vi "Accelerometer.vi"() -> ()   [LabVIEW 2021]
uses:
  <vilib>/Math Plots/3D Math Plots/3D Scatter/3D Scatter XCtrl/3D Scatter.xctl
  <vilib>/Math Plots/3D Math Plots/3D Scatter/3D Scatter Datatype/3D Scatter Datatype.lvclass
  <vilib>/DAQmx/read.llb/DAQmx Read (Analog 1D Wfm NChan NSamp).vi
  <vilib>/DAQmx/create/channels.llb/DAQmx Create Channel (AI-Voltage-Basic).vi
  <vilib>/DAQmx/configure/timing.llb/DAQmx Timing (Sample Clock).vi
  <vilib>/DAQmx/miscellaneous.llb/DAQmx Fill In Error Info.vi
  <vilib>/Utility/file.llb/Read Delimited Spreadsheet (DBL).vi
  <vilib>/Math Plots/3D Math Plots/3D Scatter/3D Scatter Datatype/Public/Plot Helper (Matrices).vi
  <vilib>/Utility/file.llb/Write Delimited Spreadsheet (DBL).vi
  <resource>/objmgr/daqmx.rc
  <vilib>/ptbypt/NI_PtbyPt.lvlib
  <vilib>/Analysis/NI_AALPro.lvlib
panel:
  out "VOLTAGE Z":dbl=-1.4400705579380926 format="%#_13g"
  in  "STOP ALL":bool
  in  "timeout":dbl=10.0 format="%0.2f"
  out "VOLTAGE Y":dbl=-1.6616253135787673 format="%#_13g"
  out "VOLTAGE X":dbl=1.114440988590271 format="%#_13g"
  out "3-Signal Waveform":waveform(dbl)[](graph)=[{"t0"=timestamp(3794378282.2177434 s since 1904-01-01), "dt"=0.001, "Y"=[1.02776641981038, 1.0481604359938839, 1.02776641981038, 1.1195394926361484, 1.1093424845443955, 1.1297365007278994, 1.1195394926361484, 1.134835004773775, 1.0991454764526445, 1.0991454764526445, 1.1705245330949072, 1.1909185492784111, 1.1654260290490317, 1.1705245330949072, 1.211312565461915, 1.1858200452325356, 1.1756230371407845, 1.1297365007278994, 1.0889484683608917, 1.0736529562232633, 0.9818798833974949, 1.0022738995809988, 1.0481604359938839, 1.114440988590271, 1.1399335088196523, 1.134835004773775, 1.1195394926361484, 1.124637996682024, 1.134835004773775, 1.0838499643150161, 1.124637996682024, 1.1450320128655278, 1.1399335088196523, 1.1603275250031562, 1.1093424845443955, 1.1501305169114033, 1.1858200452325356, 1.1399335088196523, 1.1450320128655278, 1.1450320128655278, 1.1501305169114033, 1.201115557370164, 1.201115557370164, 1.1399335088196523, 1.0991454764526445, 1.0991454764526445, 1.0940469724067672, 1.0991454764526445, 1.0838499643150161, 1.1195394926361484, 1.1195394926361484, 1.1399335088196523, 1.1552290209572806, 1.1705245330949072, 1.0991454764526445, 1.1399335088196523, 1.1501305169114033, 1.10424398049852, 1.0481604359938839, 1.0736529562232633, 1.1093424845443955, 1.1297365007278994, 1.0838499643150161, 1.058357444085635, 1.0481604359938839, 1.0532589400397594, 1.0736529562232633, 1.1195394926361484, 1.124637996682024, 1.10424398049852, 1.1399335088196523, 1.134835004773775, 1.1705245330949072, 1.1399335088196523, 1.2062140614160395, 1.1909185492784111, 1.1705245330949072, 1.1399335088196523, 1.0838499643150161, 1.124637996682024, 1.1195394926361484, 1.134835004773775, 1.0787514602691388, 1.114440988590271, 1.1399335088196523, 1.114440988590271, 1.1297365007278994, 1.0991454764526445, 1.1501305169114033, 1.134835004773775, 1.124637996682024, 1.0736529562232633, 1.0991454764526445, 1.1450320128655278, 1.1297365007278994, 1.1756230371407845, 1.1450320128655278, 1.1450320128655278, 1.114440988590271, 1.114440988590271], "attributes"=variant("NI_ChannelName"=variant(string "Dev1/ai0"), "NI_UnitDescription"=variant(string "Volts"))}, {"t0"=timestamp(3794378282.217764 s since 1904-01-01), "dt"=0.001, "Y"=[-1.6157110871262397, -1.6514221521448729, -1.6463205714279248, -1.6412189907109767, -1.6412189907109767, -1.6106095064092916, -1.6106095064092916, -1.5800000221076065, -1.5544921185228695, -1.564695279956764, -1.6055079256923452, -1.6412189907109767, -1.6412189907109767, -1.6055079256923452, -1.6106095064092916, -1.6004063449753971, -1.6055079256923452, -1.6157110871262397, -1.6208126678431878, -1.6259142485601341, -1.6004063449753971, -1.564695279956764, -1.595304764258449, -1.6412189907109767, -1.6616253135787673, -1.6463205714279248, -1.6259142485601341, -1.6055079256923452, -1.5800000221076065, -1.595304764258449, -1.5493905378059214, -1.6718284750126635, -1.6514221521448729, -1.6463205714279248, -1.6361174099940303, -1.6514221521448729, -1.73814902433298, -1.7024379593143486, -1.6973363785974005, -1.682031636446558, -1.6922347978804524, -1.6463205714279248, -1.6667268942957154, -1.6973363785974005, -1.687133217163506, -1.6769300557296098, -1.6004063449753971, -1.5851016028245546, -1.682031636446558, -1.6310158292770822, -1.595304764258449, -1.6208126678431878, -1.6106095064092916, -1.6412189907109767, -1.6106095064092916, -1.595304764258449, -1.6259142485601341, -1.6616253135787673, -1.6922347978804524, -1.6616253135787673, -1.6463205714279248, -1.687133217163506, -1.6973363785974005, -1.6769300557296098, -1.656523732861821, -1.6514221521448729, -1.6259142485601341, -1.5851016028245546, -1.6208126678431878, -1.6463205714279248, -1.595304764258449, -1.6259142485601341, -1.6922347978804524, -1.707539540031295, -1.712641120748243, -1.6667268942957154, -1.6973363785974005, -1.682031636446558, -1.7177427014651911, -1.6718284750126635, -1.687133217163506, -1.7432506050499281, -1.73814902433298, -1.6973363785974005, -1.6973363785974005, -1.682031636446558, -1.6514221521448729, -1.6361174099940303, -1.5851016028245546, -1.6208126678431878, -1.5800000221076065, -1.595304764258449, -1.6106095064092916, -1.569796860673712, -1.5851016028245546, -1.564695279956764, -1.5748984413906602, -1.6004063449753971, -1.6514221521448729, -1.6616253135787673], "attributes"=variant("NI_ChannelName"=variant(string "Dev1/ai1"), "NI_UnitDescription"=variant(string "Volts"))}, {"t0"=timestamp(3794378282.217785 s since 1904-01-01), "dt"=0.001, "Y"=[-1.3533473747749927, -1.3584487384904698, -1.3788541933523764, -1.3329419199130879, -1.2972323739047518, -1.307435101335706, -1.2972323739047518, -1.276826919042847, -1.3329419199130879, -1.3788541933523764, -1.3890569207833288, -1.3023337376202289, -1.338043283628565, -1.4400705579380926, -1.4400705579380926, -1.4400705579380926, -1.4400705579380926, -1.4247664667916649, -1.3992596482142812, -1.4196651030761878, -1.4604760127999992, -1.5063882862392877, -1.4910841950928582, -1.4655773765154763, -1.485982831377381, -1.4961855588083353, -1.455374649084522, -1.3890569207833288, -1.3329419199130879, -1.3788541933523764, -1.3788541933523764, -1.4808814676619058, -1.3584487384904698, -1.3431446473440403, -1.3533473747749927, -1.2717255553273699, -1.2411173730345109, -1.338043283628565, -1.3839555570678517, -1.338043283628565, -1.4451719216535697, -1.3941582844988059, -1.338043283628565, -1.4196651030761878, -1.4349691942226173, -1.3737528296368993, -1.3584487384904698, -1.3176378287666584, -1.4910841950928582, -1.3992596482142812, -1.3176378287666584, -1.3584487384904698, -1.2564214641809404, -1.3533473747749927, -1.3635501022059469, -1.3329419199130879, -1.338043283628565, -1.3635501022059469, -1.3584487384904698, -1.3584487384904698, -1.3125364650511813, -1.307435101335706, -1.3278405561976108, -1.3737528296368993, -1.3890569207833288, -1.338043283628565, -1.3125364650511813, -1.3533473747749927, -1.4298678305071402, -1.4604760127999992, -1.3992596482142812, -1.4349691942226173, -1.3737528296368993, -1.3941582844988059, -1.4094623756452354, -1.4298678305071402, -1.4757801039464287, -1.455374649084522, -1.4961855588083353, -1.4400705579380926, -1.4604760127999992, -1.4808814676619058, -1.5012869225238106, -1.4451719216535697, -1.5012869225238106, -1.5523005596785762, -1.4655773765154763, -1.3890569207833288, -1.3737528296368993, -1.4808814676619058, -1.4655773765154763, -1.5676046508250057, -1.4706787402309516, -1.485982831377381, -1.4094623756452354, -1.3737528296368993, -1.4043610119297583, -1.4451719216535697, -1.4400705579380926, -1.4400705579380926], "attributes"=variant("NI_ChannelName"=variant(string "Dev1/ai2"), "NI_UnitDescription"=variant(string "Volts"))}]
  out "Z-Signal Waveform":dynamicdata(graph)=[{"t0"=timestamp(3794378282.217785 s since 1904-01-01), "dt"=0.001, "Y"=[-1.3533473747749927, -1.3584487384904698, -1.3788541933523764, -1.3329419199130879, -1.2972323739047518, -1.307435101335706, -1.2972323739047518, -1.276826919042847, -1.3329419199130879, -1.3788541933523764, -1.3890569207833288, -1.3023337376202289, -1.338043283628565, -1.4400705579380926, -1.4400705579380926, -1.4400705579380926, -1.4400705579380926, -1.4247664667916649, -1.3992596482142812, -1.4196651030761878, -1.4604760127999992, -1.5063882862392877, -1.4910841950928582, -1.4655773765154763, -1.485982831377381, -1.4961855588083353, -1.455374649084522, -1.3890569207833288, -1.3329419199130879, -1.3788541933523764, -1.3788541933523764, -1.4808814676619058, -1.3584487384904698, -1.3431446473440403, -1.3533473747749927, -1.2717255553273699, -1.2411173730345109, -1.338043283628565, -1.3839555570678517, -1.338043283628565, -1.4451719216535697, -1.3941582844988059, -1.338043283628565, -1.4196651030761878, -1.4349691942226173, -1.3737528296368993, -1.3584487384904698, -1.3176378287666584, -1.4910841950928582, -1.3992596482142812, -1.3176378287666584, -1.3584487384904698, -1.2564214641809404, -1.3533473747749927, -1.3635501022059469, -1.3329419199130879, -1.338043283628565, -1.3635501022059469, -1.3584487384904698, -1.3584487384904698, -1.3125364650511813, -1.307435101335706, -1.3278405561976108, -1.3737528296368993, -1.3890569207833288, -1.338043283628565, -1.3125364650511813, -1.3533473747749927, -1.4298678305071402, -1.4604760127999992, -1.3992596482142812, -1.4349691942226173, -1.3737528296368993, -1.3941582844988059, -1.4094623756452354, -1.4298678305071402, -1.4757801039464287, -1.455374649084522, -1.4961855588083353, -1.4400705579380926, -1.4604760127999992, -1.4808814676619058, -1.5012869225238106, -1.4451719216535697, -1.5012869225238106, -1.5523005596785762, -1.4655773765154763, -1.3890569207833288, -1.3737528296368993, -1.4808814676619058, -1.4655773765154763, -1.5676046508250057, -1.4706787402309516, -1.485982831377381, -1.4094623756452354, -1.3737528296368993, -1.4043610119297583, -1.4451719216535697, -1.4400705579380926, -1.4400705579380926], "attributes"=variant("NI_ChannelName"=variant(string "Dev1/ai2"), "NI_UnitDescription"=variant(string "Volts"))}]
  out "Y-Signal Waveform":dynamicdata(graph)=[{"t0"=timestamp(3794378282.217764 s since 1904-01-01), "dt"=0.001, "Y"=[-1.6157110871262397, -1.6514221521448729, -1.6463205714279248, -1.6412189907109767, -1.6412189907109767, -1.6106095064092916, -1.6106095064092916, -1.5800000221076065, -1.5544921185228695, -1.564695279956764, -1.6055079256923452, -1.6412189907109767, -1.6412189907109767, -1.6055079256923452, -1.6106095064092916, -1.6004063449753971, -1.6055079256923452, -1.6157110871262397, -1.6208126678431878, -1.6259142485601341, -1.6004063449753971, -1.564695279956764, -1.595304764258449, -1.6412189907109767, -1.6616253135787673, -1.6463205714279248, -1.6259142485601341, -1.6055079256923452, -1.5800000221076065, -1.595304764258449, -1.5493905378059214, -1.6718284750126635, -1.6514221521448729, -1.6463205714279248, -1.6361174099940303, -1.6514221521448729, -1.73814902433298, -1.7024379593143486, -1.6973363785974005, -1.682031636446558, -1.6922347978804524, -1.6463205714279248, -1.6667268942957154, -1.6973363785974005, -1.687133217163506, -1.6769300557296098, -1.6004063449753971, -1.5851016028245546, -1.682031636446558, -1.6310158292770822, -1.595304764258449, -1.6208126678431878, -1.6106095064092916, -1.6412189907109767, -1.6106095064092916, -1.595304764258449, -1.6259142485601341, -1.6616253135787673, -1.6922347978804524, -1.6616253135787673, -1.6463205714279248, -1.687133217163506, -1.6973363785974005, -1.6769300557296098, -1.656523732861821, -1.6514221521448729, -1.6259142485601341, -1.5851016028245546, -1.6208126678431878, -1.6463205714279248, -1.595304764258449, -1.6259142485601341, -1.6922347978804524, -1.707539540031295, -1.712641120748243, -1.6667268942957154, -1.6973363785974005, -1.682031636446558, -1.7177427014651911, -1.6718284750126635, -1.687133217163506, -1.7432506050499281, -1.73814902433298, -1.6973363785974005, -1.6973363785974005, -1.682031636446558, -1.6514221521448729, -1.6361174099940303, -1.5851016028245546, -1.6208126678431878, -1.5800000221076065, -1.595304764258449, -1.6106095064092916, -1.569796860673712, -1.5851016028245546, -1.564695279956764, -1.5748984413906602, -1.6004063449753971, -1.6514221521448729, -1.6616253135787673], "attributes"=variant("NI_ChannelName"=variant(string "Dev1/ai1"), "NI_UnitDescription"=variant(string "Volts"))}]
  out "X-Signal Waveform":dynamicdata(graph)=[{"t0"=timestamp(3794378282.2177434 s since 1904-01-01), "dt"=0.001, "Y"=[1.02776641981038, 1.0481604359938839, 1.02776641981038, 1.1195394926361484, 1.1093424845443955, 1.1297365007278994, 1.1195394926361484, 1.134835004773775, 1.0991454764526445, 1.0991454764526445, 1.1705245330949072, 1.1909185492784111, 1.1654260290490317, 1.1705245330949072, 1.211312565461915, 1.1858200452325356, 1.1756230371407845, 1.1297365007278994, 1.0889484683608917, 1.0736529562232633, 0.9818798833974949, 1.0022738995809988, 1.0481604359938839, 1.114440988590271, 1.1399335088196523, 1.134835004773775, 1.1195394926361484, 1.124637996682024, 1.134835004773775, 1.0838499643150161, 1.124637996682024, 1.1450320128655278, 1.1399335088196523, 1.1603275250031562, 1.1093424845443955, 1.1501305169114033, 1.1858200452325356, 1.1399335088196523, 1.1450320128655278, 1.1450320128655278, 1.1501305169114033, 1.201115557370164, 1.201115557370164, 1.1399335088196523, 1.0991454764526445, 1.0991454764526445, 1.0940469724067672, 1.0991454764526445, 1.0838499643150161, 1.1195394926361484, 1.1195394926361484, 1.1399335088196523, 1.1552290209572806, 1.1705245330949072, 1.0991454764526445, 1.1399335088196523, 1.1501305169114033, 1.10424398049852, 1.0481604359938839, 1.0736529562232633, 1.1093424845443955, 1.1297365007278994, 1.0838499643150161, 1.058357444085635, 1.0481604359938839, 1.0532589400397594, 1.0736529562232633, 1.1195394926361484, 1.124637996682024, 1.10424398049852, 1.1399335088196523, 1.134835004773775, 1.1705245330949072, 1.1399335088196523, 1.2062140614160395, 1.1909185492784111, 1.1705245330949072, 1.1399335088196523, 1.0838499643150161, 1.124637996682024, 1.1195394926361484, 1.134835004773775, 1.0787514602691388, 1.114440988590271, 1.1399335088196523, 1.114440988590271, 1.1297365007278994, 1.0991454764526445, 1.1501305169114033, 1.134835004773775, 1.124637996682024, 1.0736529562232633, 1.0991454764526445, 1.1450320128655278, 1.1297365007278994, 1.1756230371407845, 1.1450320128655278, 1.1450320128655278, 1.114440988590271, 1.114440988590271], "attributes"=variant("NI_ChannelName"=variant(string "Dev1/ai0"), "NI_UnitDescription"=variant(string "Volts"))}]
  out "SampClk.Rate":dbl=1000.0
  in  "Modalità di campionamento":i32(ring)=10123 items=["Finite Samples"=10178, "Continuous Samples"=10123, "Hardware Timed Single Point"=12522]
  in  "Campioni per canale":i32=100
  in  "Rate":dbl=1000.0 format="%0.2f"
  in  "Canale Fisico":tag="Dev1/ai0:2"
  in  "MIN Value":dbl=-10.0 format="%0.2f"
  in  "MAX Value":dbl=10.0 format="%0.2f"
  in  "Tab Control":T1(tab)=enum."CALIBRATION"
  in  "File z":path=path "C:/Users/Engel/Desktop/MAIP_Project/Z.csv"
  in  "File y":path=path "C:/Users/Engel/Desktop/MAIP_Project/Y.csv"
  in  "File x":path=path "C:/Users/Engel/Desktop/MAIP_Project/X.csv"
  in  "Salvare su file?":bool=TRUE
  out "Real values":refnum<class "3D Plot Datatype.lvclass">[](xcontrol)
  in  "Usare il filtro a\n media mobile?":bool
  out "h":dbl[][](array[numeric])
  in  "Z":path=path "C:/Users/Engel/Documents/Dati_ellisse/dati_buoni_BRACCIO/Z.csv"
  in  "X":path=path "C:/Users/Engel/Documents/Dati_ellisse/dati_buoni_BRACCIO/X.csv"
  in  "Y":path=path "C:/Users/Engel/Documents/Dati_ellisse/dati_buoni_BRACCIO/Y.csv"
  out "Real values 2":refnum<class "3D Plot Datatype.lvclass">[](xcontrol)
  out "Best Linear Fit":dbl[](array[numeric])=[-90.70772285582407, 1.4505193173588147, 89.25720353846528]
  in  "Tensioni":path=path "C:/Users/Engel/Desktop/Dati/Z TAR/mean_z.txt"
  in  "Gradi":path=path "C:/Users/Engel/Desktop/Dati/Gradi6/Gradi.txt"
  out "Gradi\nz":dbl[](array[numeric])=[-91.51190382332419]
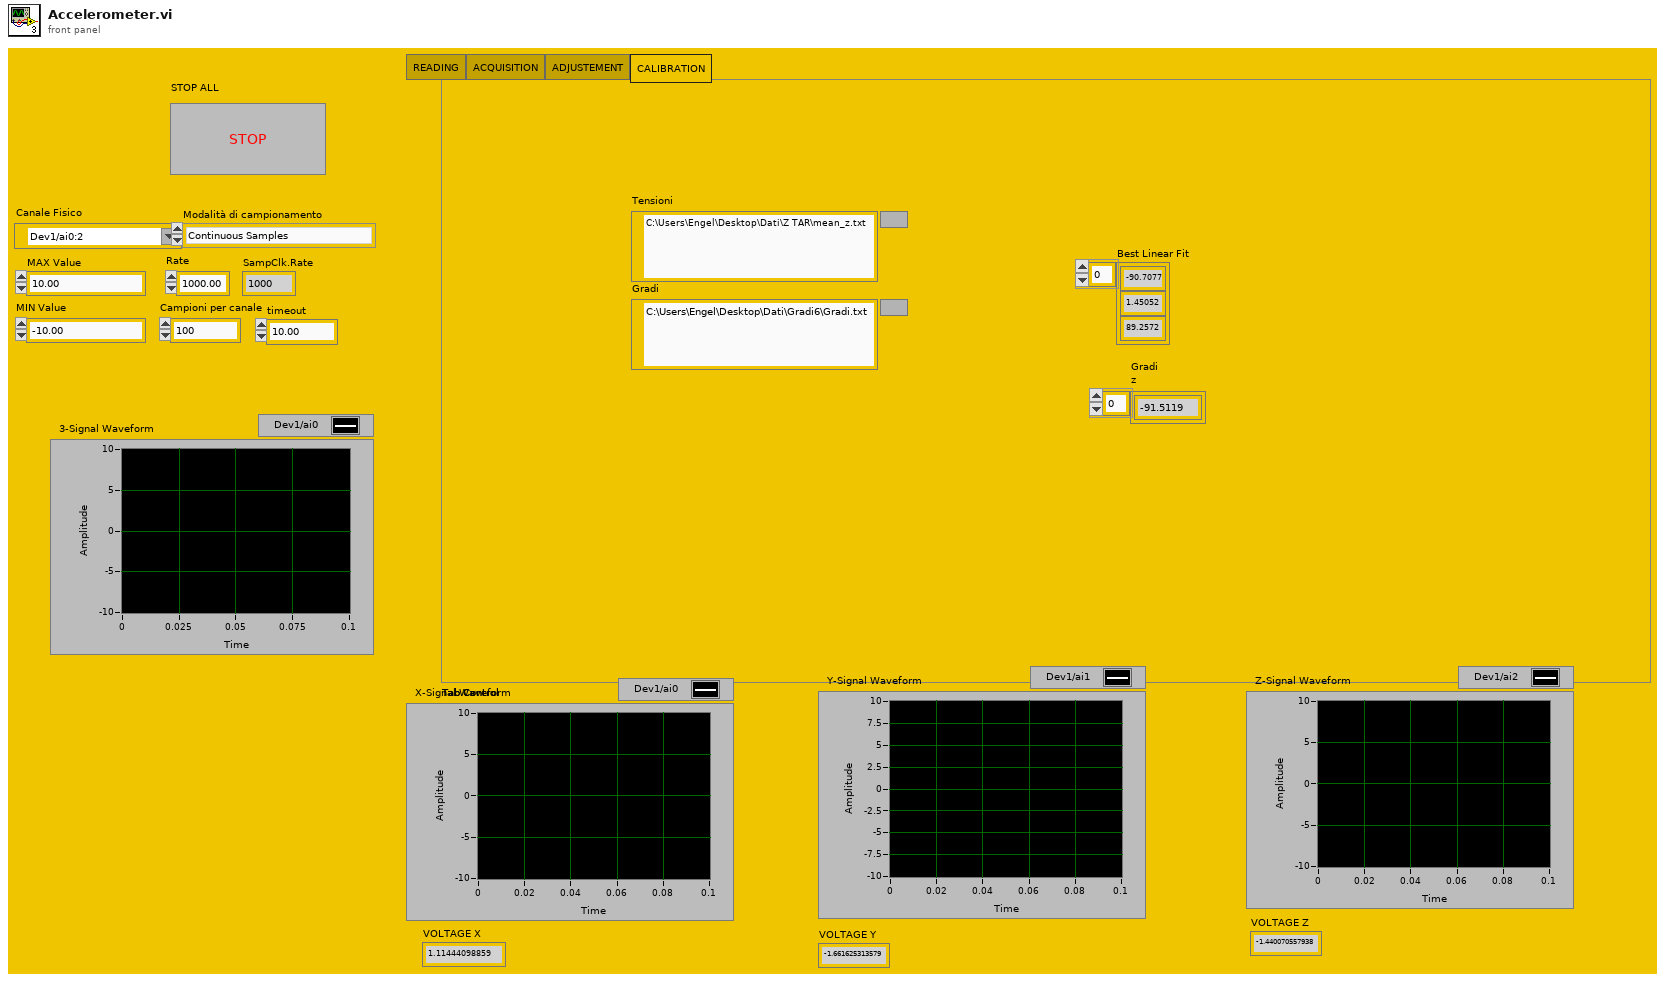
[diagram p1: front panel]
types:
  T1 = enum32{"READING", "ACQUISITION", "ADJUSTEMENT", "CALIBRATION"}
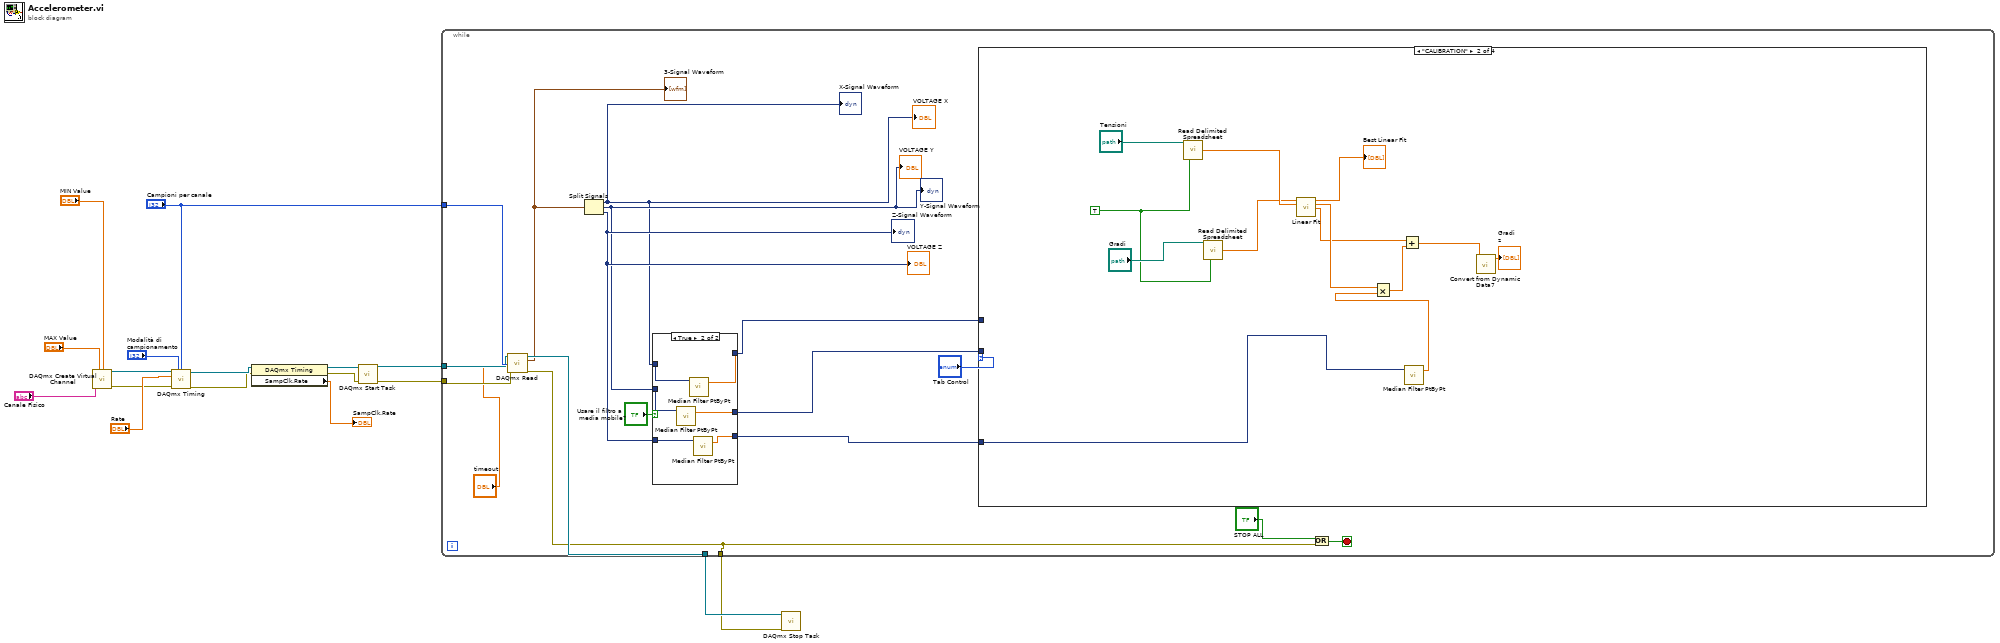
[diagram p0: block diagram]
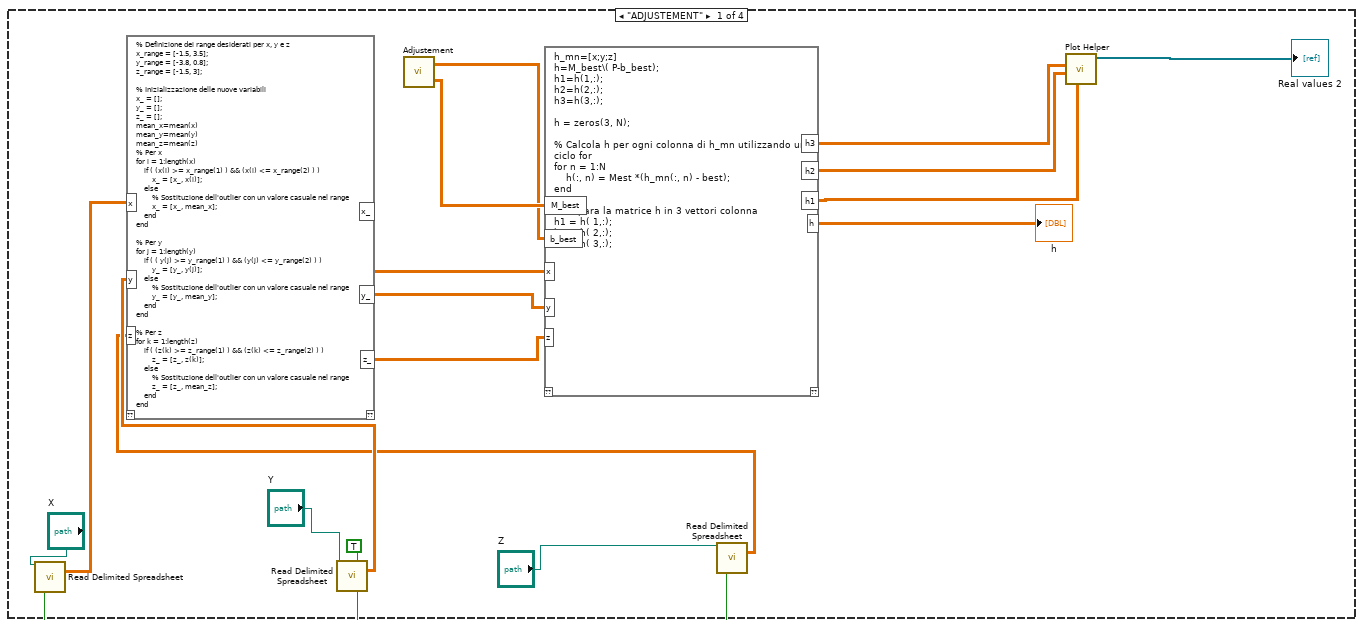
[diagram p3: hidden frame]
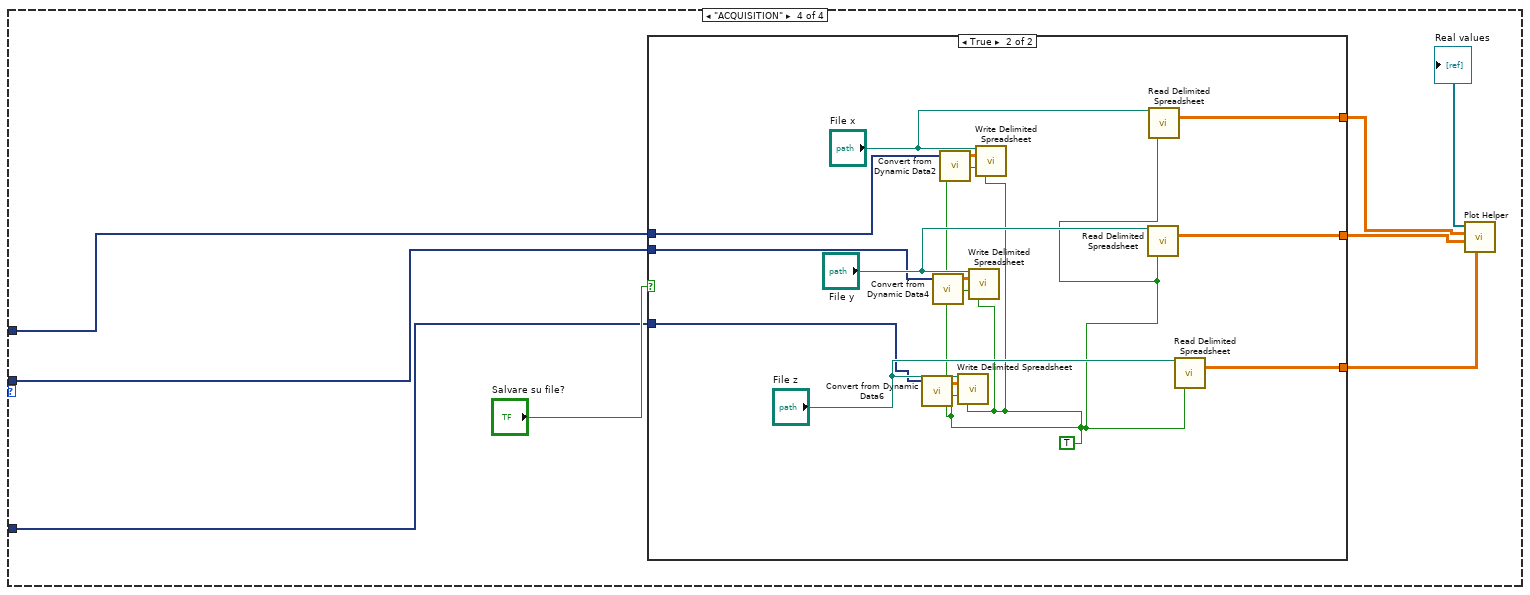
[diagram p5: hidden frame]
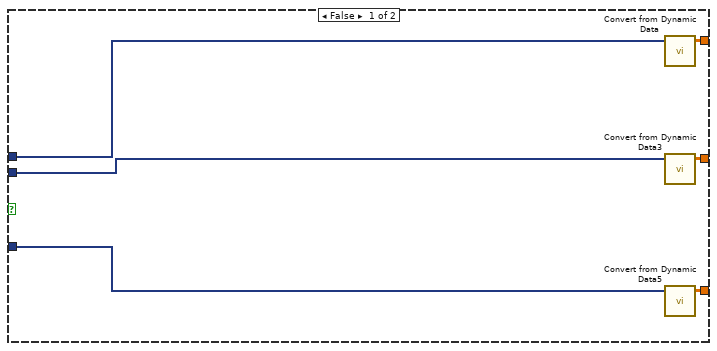
[diagram p6: hidden frame]
diagram:
  n1 = call-poly <vilib>:"DAQmx Create Virtual Channel.vi"("maximum value"="MAX Value", "minimum value"="MIN Value", "physical channels"="Canale Fisico") -> ("task out"=w14:refnum<k21>, "error out"=w11:errorcluster)  [unwired: 11 in]
  n2 = call-poly <vilib>:"DAQmx Timing.vi"("task/channels in"=w14, "sample mode"="Modalità di campionamento", "samples per channel"="Campioni per canale", "rate"="Rate", "error in"=w11) -> ("task out"=w9:refnum<k21>, "error out"=w8:errorcluster)  [unwired: 9 in]
  n3 = property class="DAQmx Timing"(reference=w9, error in=w8) -> (reference out=w7:refnum<k21>, error out=w6:errorcluster, "SampClk.Rate"=→"SampClk.Rate":dbl)
  n4 = call <vilib>:"DAQmx Start Task.vi"("task/channels in"=w7, "error in"=w6) -> ("task out"=w5:refnum<k21>, "error out"=w3:errorcluster)  [unwired: 12 in]
  n5 = while {
    tunnel: w5 -> [w30]
    tunnel: "Campioni per canale" -> [w31]
    tunnel: w3 -> [w29]
    tunnel: [w28] -> w2
    tunnel: [w27] -> w1
    stop <- w32 stop-if-true
    n6 = call-poly <vilib>:"DAQmx Read.vi"("task/channels in"=w30, "number of samples per channel"=w31, "timeout"="timeout", "error in"=w29) -> ("task out"=w28:refnum<k21>, "data"=w26:waveform(dbl)[], "error out"=w27:errorcluster)  [unwired: 9 in]
    "3-Signal Waveform" <- w26
    n7 = Split Signals(w26) -> (w20:dynamicdata, w22:dynamicdata, w24:dynamicdata)  [unwired: 3 in]
    "Z-Signal Waveform" <- w24
    "Y-Signal Waveform" <- w22
    "X-Signal Waveform" <- w20
    "VOLTAGE X" <- w20
    "VOLTAGE Y" <- w22
    "VOLTAGE Z" <- w24
    n8 = case shown="True" "Usare il filtro a\n media mobile?" {
      tunnel: w24 -> [w35 w43]
      tunnel: [w35 w42] -> w23
      tunnel: w22 -> [w36 w41]
      tunnel: [w36 w40] -> w21
      tunnel: w20 -> [w37 w39]
      tunnel: [w37 w38] -> w19
      frame False {
      }
      frame True {
        n9 = call <vilib>:"Median Filter PtByPt.vi"("x"=w41) -> ("Filtered x"=w40:dbl)  [unwired: 3 in, 1 out]
        n10 = call <vilib>:"Median Filter PtByPt.vi"("x"=w39) -> ("Filtered x"=w38:dbl)  [unwired: 3 in, 1 out]
        n11 = call <vilib>:"Median Filter PtByPt.vi"("x"=w43) -> ("Filtered x"=w42:dbl)  [unwired: 3 in, 1 out]
      }
    }
    n12 = case shown="\"CALIBRATION\"" "Tab Control" {
      tunnel: w19 -> [_ _ _ w76]
      tunnel: w21 -> [_ _ _ w75]
      tunnel: w23 -> [_ w62 _ w74]
      frame "ADJUSTEMENT" {
        w55 = TRUE ("transpose? (F)")
        n13 = call-poly <vilib>:"Read Delimited Spreadsheet.vi"("file path (dialog if empty)"="X", "transpose? (F)"=w55) -> ("all rows"=w49:dbl[][])  [unwired: 8 in, 5 out]
        n14 = call-poly <vilib>:"Read Delimited Spreadsheet.vi"("file path (dialog if empty)"="Y", "transpose? (F)"=w55) -> ("all rows"=w48:dbl[][])  [unwired: 8 in, 5 out]
        n15 = call "Adjustement.vi"() -> ("M_best"=w51:dbl[][], "B"=w50:dbl[][])  [unwired: 2 in]
        n16 = call-poly <vilib>:"Read Delimited Spreadsheet.vi"("file path (dialog if empty)"="Z", "transpose? (F)"=w55) -> ("all rows"=w47:dbl[][])  [unwired: 8 in, 5 out]
        n17 = script code="% Definizione dei range desiderati per x, y e z\nx_range = [-1.5, 3.5];\ny_range = [-3.8, 0.8];\nz_range = [-1.5, 3];\n\n% Inizializzazione delle nuove variabili\nx_ = [];\ny_ = [];\nz_ = [];\nmean_x=mean(x)\nmean_y=mean(y)\nmean_z=mean(z)\n% Per x\nfor i = 1:length(x)\n    if ( (x(i) >= x_range(1) ) && (x(i) <= x_range(2) ) )\n        x_ = [x_, x(i)];\n    else\n        % Sostituzione dell'outlier con un valore casuale nel range\n        x_ = [x_, mean_x];\n    end\nend\n\n% Per y\nfor j = 1:length(y)\n    if ( ( y(j) >= y_range(1) ) && (y(j) <= y_range(2) ) )\n        y_ = [y_, y(j)];\n    else\n        % Sostituzione dell'outlier con un valore casuale nel range\n        y_ = [y_, mean_y];\n    end\nend\n\n% Per z\nfor k = 1:length(z)\n    if ( (z(k) >= z_range(1) ) && (z(k) <= z_range(2) ) )\n        z_ = [z_, z(k)];\n    else\n        % Sostituzione dell'outlier con un valore casuale nel range\n        z_ = [z_, mean_z];\n    end\nend"("x"=w49, "y"=w48, "z"=w47) -> ("x_"=w46:dbl[][], "y_"=w45:dbl[][], "z_"=w44:dbl[][])  [unwired: 1 in, 1 out]
        n18 = script code="h_mn=[x;y;z]\nh=M_best\\( P-b_best);\nh1=h(1,:);\nh2=h(2,:);\nh3=h(3,:);\n\nh = zeros(3, N);\n\n% Calcola h per ogni colonna di h_mn utilizzando un ciclo for\nfor n = 1:N\n    h(:, n) = Mest *(h_mn(:, n) - best);\nend\n\n% Separa la matrice h in 3 vettori colonna\nh1 = h( 1,:);\nh2 = h( 2,:);\nh3 = h( 3,:);"("M_best"=w51, "b_best"=w50, "x"=w46, "y"=w45, "z"=w44) -> ("h"=→"h":dbl[][], "h1"=w52:dbl[][], "h2"=w53:dbl[][], "h3"=w54:dbl[][])  [unwired: 1 in, 1 out]
        n19 = call-poly <vilib>:"Plot Helper.vi"("z matrix"=w52, "y matrix"=w53, "x matrix"=w54) -> ("3D Plot lvclass Array out"=→"Real values 2":refnum<class "3D Plot Datatype.lvclass">[])  [unwired: 3 in, 5 out]
      }
      frame "CALIBRATION" {
        w69 = TRUE ("transpose? (F)")
        n20 = call-poly <vilib>:"Read Delimited Spreadsheet.vi"("file path (dialog if empty)"="Tensioni", "transpose? (F)"=w69) -> ("first row"=w71:dbl[])  [unwired: 8 in, 5 out]
        n21 = call-poly <vilib>:"Read Delimited Spreadsheet.vi"("file path (dialog if empty)"="Gradi", "transpose? (F)"=w69) -> ("first row"=w70:dbl[])  [unwired: 8 in, 5 out]
        n22 = call <vilib>:"Linear Fit.vi"("Y"=w70, "X"=w71) -> ("Best Linear Fit"=→"Best Linear Fit":dbl[], "slope"=w67:dbl, "intercept"=w66:dbl)  [unwired: 9 in, 2 out]
        n23 = call <vilib>:"Median Filter PtByPt.vi"("x"=w62) -> ("Filtered x"=w61:dbl)  [unwired: 3 in, 1 out]
        n24 = Multiply(x=w67, y=w61) -> (x*y=w65:dbl)
        n25 = Add(x=w66, y=w65) -> (x+y=w64:dbl)
        n26 = call "Convert from Dynamic Data7"("Dynamic Data Type"=w64) -> ("Array"=→"Gradi\nz":dbl[])  [unwired: 3 in]
      }
      frame "READING", Default {
      }
      frame "ACQUISITION" {
        n27 = case shown="True" "Salvare su file?" {
          tunnel: w76 -> [w87 w93]
          tunnel: w75 -> [w86 w91]
          tunnel: w74 -> [w85 w92]
          tunnel: [w82 w97] -> w80
          tunnel: [w83 w96] -> w79
          tunnel: [w84 w95] -> w78
          frame False {
            n28 = call "Convert from Dynamic Data"("Dynamic Data Type"=w87) -> ("Array"=w84:dbl[][])  [unwired: 3 in]
            n29 = call "Convert from Dynamic Data3"("Dynamic Data Type"=w86) -> ("Array"=w83:dbl[][])  [unwired: 3 in]
            n30 = call "Convert from Dynamic Data5"("Dynamic Data Type"=w85) -> ("Array"=w82:dbl[][])  [unwired: 3 in]
          }
          frame True {
            w94 = TRUE
            n31 = call "Convert from Dynamic Data6"("Dynamic Data Type"=w92) -> ("Array"=w88:dbl[][])  [unwired: 3 in]
            n32 = call "Convert from Dynamic Data4"("Dynamic Data Type"=w91) -> ("Array"=w89:dbl[][])  [unwired: 3 in]
            n33 = call "Convert from Dynamic Data2"("Dynamic Data Type"=w93) -> ("Array"=w90:dbl[][])  [unwired: 3 in]
            n34 = call-poly <vilib>:"Write Delimited Spreadsheet.vi"("file path (dialog if empty)"="File z", "2D data"=w88, "append to file? (new file:F)"=w94, "transpose? (no:F)"=w94) -> ()  [unwired: 10 in, 2 out]
            n35 = call-poly <vilib>:"Write Delimited Spreadsheet.vi"("file path (dialog if empty)"="File y", "2D data"=w89, "append to file? (new file:F)"=w94, "transpose? (no:F)"=w94) -> ()  [unwired: 10 in, 2 out]
            n36 = call-poly <vilib>:"Write Delimited Spreadsheet.vi"("file path (dialog if empty)"="File x", "2D data"=w90, "append to file? (new file:F)"=w94, "transpose? (no:F)"=w94) -> ()  [unwired: 10 in, 2 out]
            n37 = call-poly <vilib>:"Read Delimited Spreadsheet.vi"("file path (dialog if empty)"="File y", "transpose? (F)"=w94) -> ("all rows"=w96:dbl[][])  [unwired: 8 in, 5 out]
            n38 = call-poly <vilib>:"Read Delimited Spreadsheet.vi"("file path (dialog if empty)"="File x", "transpose? (F)"=w94) -> ("all rows"=w95:dbl[][])  [unwired: 8 in, 5 out]
            n39 = call-poly <vilib>:"Read Delimited Spreadsheet.vi"("file path (dialog if empty)"="File z", "transpose? (F)"=w94) -> ("all rows"=w97:dbl[][])  [unwired: 8 in, 5 out]
          }
        }
        n40 = call-poly <vilib>:"Plot Helper.vi"("z matrix"=w80, "y matrix"=w79, "x matrix"=w78) -> ("3D Plot lvclass Array out"=→"Real values":refnum<class "3D Plot Datatype.lvclass">[])  [unwired: 3 in, 5 out]
      }
    }
    n41 = Or(x="STOP ALL", y=w27) -> (x .or. y?=w32:bool)
  }
  n42 = call <vilib>:"DAQmx Stop Task.vi"("task/channels in"=w2, "error in"=w1) -> ()  [unwired: 12 in, 2 out]
